vi "AAA Hacker A150-12 THRUST LEVER.vi"() -> ()   [LabVIEW 2020]
uses:
  <instrlib>/Gantner Instruments/Ethernet/Gantner-Instruments HighSpeedPort.llb/e.gate Protocol Type.ctl
  <vilib>/Utility/file.llb/Write Delimited Spreadsheet (string).vi
panel:
  out "Elapsed Time":string
  out "?":dbl[](array[slide]) scale=0.0..1000.0
  out "Temperature 2":dbl[](array[slide]) caption="Thermocouple 1" scale=20.0..50.0
  out "error out 2":errorcluster
  in  "?":bool
  # "Hacker A150-12  -  Motor control"
  # "Temperatures"
  # "Torque"
  # "Vibration"
  # "Power Supply"
  # "Atmospheric\nConditions"
  # "Voltage"
  # "Thrust"
  # "Current"
  # "Battery Data"
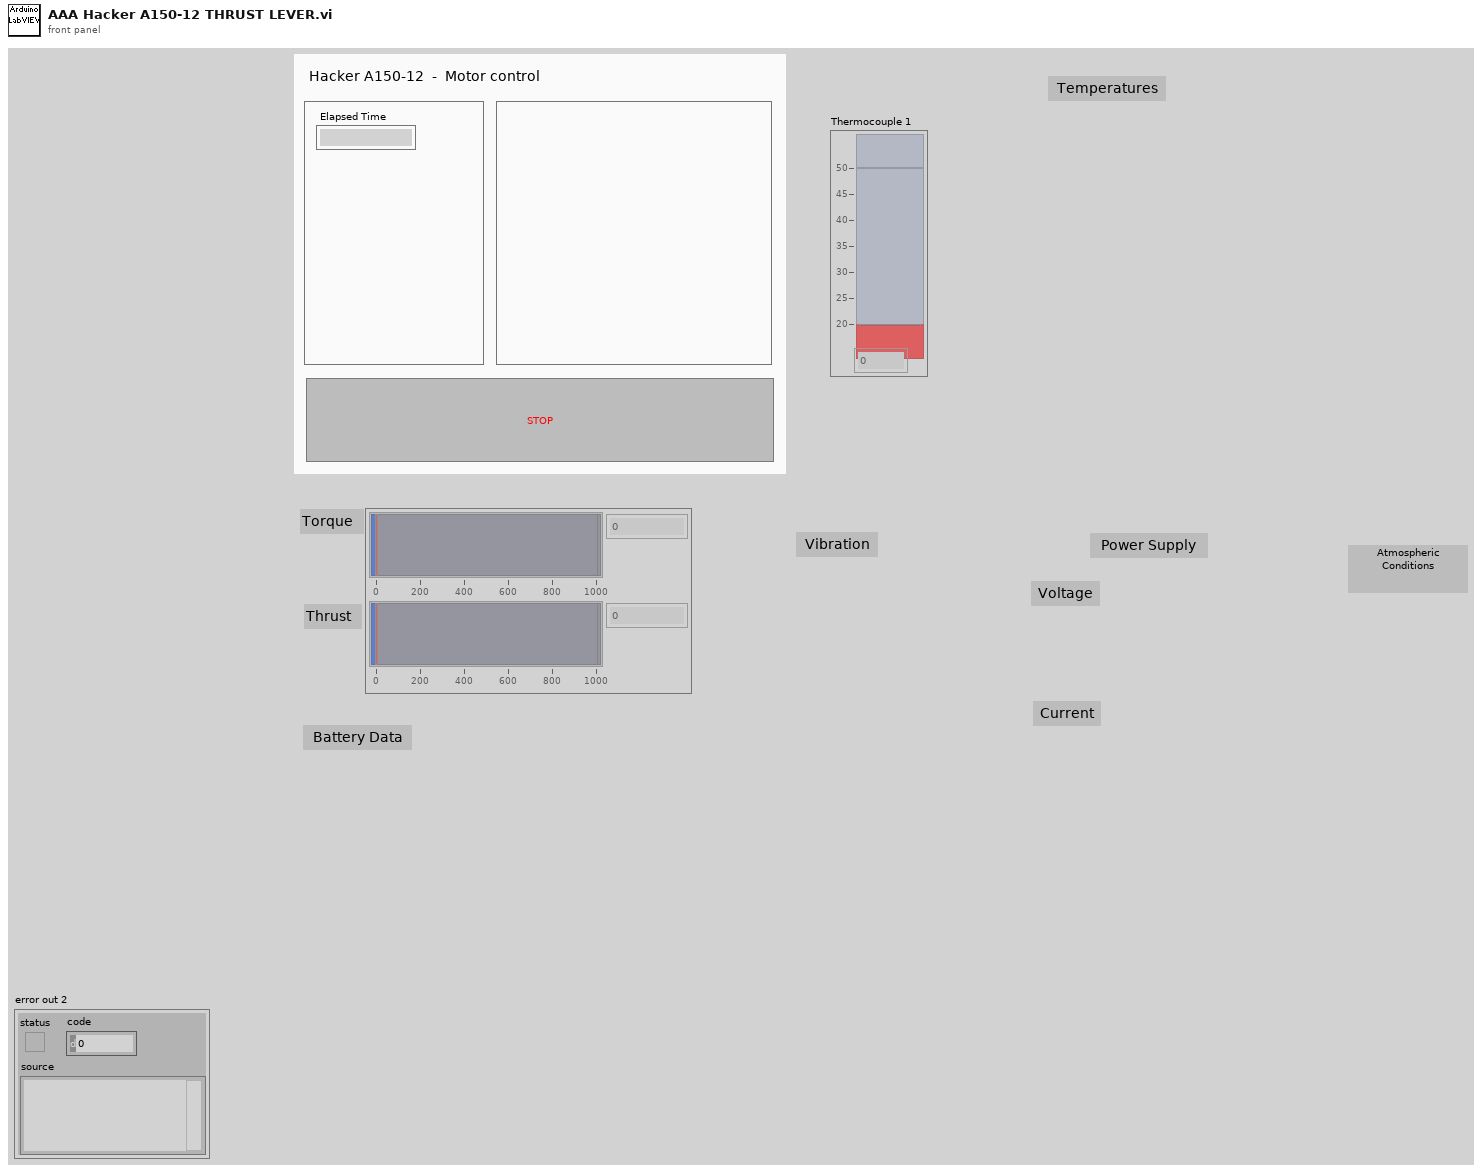
[diagram p1: front panel]
types:
  T1 = typedef "e.gate Protocol Type.ctl" = enum16{"ASCII", "HighspeedPort Online", "HighspeedPort Buffer (giutility.DLL) ", "PostProcessBuffer (giutility.DLL)", "HighspeedPort Online (giutility.DLL)", "Decode UDBF File (giutility.DLL)"}
  T2 = typedef "e.gate Configuration.ctl" = cluster{"connection ID":refnum<k5>, "IPAddress":string, "BufferIndex":i32, "StateMessage":string, "StateCode":i8, "HeaderSize":i32, "BufferSize":i32, "IsBigEndian":i32, "Version":i32, "ChannelCount":i32, "FrameLength":i32, "StartTime":dbl, "dActTimeToSecondFactor":dbl, "StartTimeToDayFactor":dbl, "BufferFillRate":dbl, "SampleRate":dbl, "ChannelData":T3[], "DecodeTimeFormat":string, "SummaryPath":string, "WithCheckSum":i32, "dActTimeDataType":T4, "MaxWriteCount":i32, "MaxReadCount":i32, "TempOffsetRead":i32, "TempLengthRead":i32, "Protocol":T1, "IsSupported":i32, "InputAccessList":i32[], "OutputAccessList":i32[], "DataSource":enum16{"CircleBuffer", "test.con Logger", "test.con Archive"}, "Modules":T5[], "DLL-Handle":T6}
  T3 = typedef "e.gate Channel Data.ctl" = cluster{"VariableName":string, "DataDirection":string, "DataType":string, "DataTypeIndex":T4, "Precision":i16, "FieldLengtht":i16, "ByteCount":i32, "Format":string, "Unit":string, "InputAccessOffset":i32, "OutputAccessOffset":i16, "InputAccessIndex":i16, "OutputAccessIndex":i16, "VarType":string}
  T4 = typedef "e.gate Data Type.ctl" = enum16{"NO", "BOOL", "SINT8", "USINT8", "SINT16", "USINT16", "SINT32", "USINT32", "FLOAT", "SET8", "SET16", "SET32", "DOUBLE", "SINT64", "USINT64", "SET64"}
  T5 = typedef "e.gate Module  Data.ctl" = cluster{"Type":string, "Location":string, "VariablesCount":i16, "UartIndex":i16, "Address":i16, "SystemOffset":i16}
  T6 = typedef "e.gateHSP_DLLhandle.ctl" = cluster{"clientInstance":i32, "connectionInstance":i32, "Is32Bit":bool, "DLL Path":path}
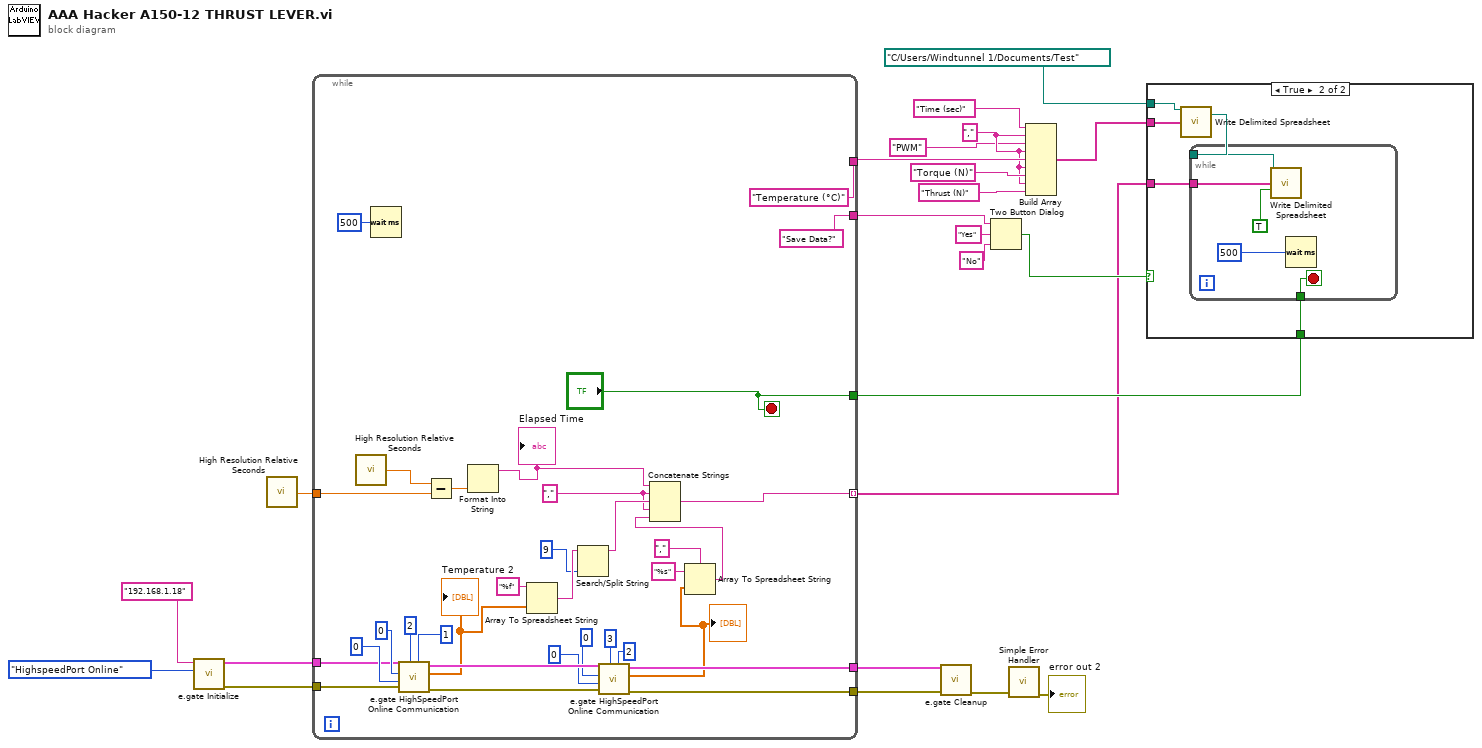
[diagram p0: block diagram]
diagram:
  w2 = "," ("element")
  n1 = call <instrlib>:"e.gate Initialize.vi"("Protocol"=e.gate_Protocol_Type."HighspeedPort Online", "IP Address"="192.168.1.18") -> ("error out"=w18:errorcluster, "e.gate Configuration"=w19:T2)  [unwired: 8 in]
  n2 = call <vilib>:"High Resolution Relative Seconds.vi"() -> ("relative seconds"=w7:dbl)
  n3 = while {
    tunnel: w19 -> [w45]
    tunnel: w18 -> [w44]
    tunnel: [w27] -> w17
    tunnel: [w43] -> w16
    tunnel: ["Save Data?" ("message")] -> w11
    tunnel: ["?"] -> w10
    tunnel: ["Temperature (°C)" ("element")] -> w9
    tunnel: w7 -> [w38]
    tunnel: [w34] -> w8 mode=indexing
    stop <- "?" stop-if-true
    w28 = "," ("string")
    n4 = call <vilib>:"High Resolution Relative Seconds.vi"() -> ("relative seconds"=w39:dbl)
    n5 = Wait (ms)(milliseconds to wait=u32 500) -> ()  [unwired: 1 out]
    n6 = call <instrlib>:"e.gate HighSpeedPort Online Communication.vi"("ReadCount"=1, "ReadIndex"=2, "error in (no error)"=w44, "WriteCount"=0, "WriteIndex"=0, "e.gate Configuration In"=w45) -> ("error out"=w50:errorcluster, "Value"=w40:dbl[], "e.gate Configuration Out"=w51:T2)  [unwired: 3 in]
    "Temperature 2" <- w40
    n7 = Subtract(x=w39, y=w38) -> (x-y=w37:dbl)
    n8 = Format Into String(w37) -> (resulting string=w25:string)  [unwired: 3 in, 1 out]
    "Elapsed Time" <- w25
    n9 = Array To Spreadsheet String(array=w40, 3:"%f" ("format string")) -> (spreadsheet string=w31:string)  [unwired: 1 in]
    n10 = Search/Split String(string=w31, offset (0)=9) -> (substring before match=w30:string)  [unwired: 1 in, 2 out]
    n11 = call <instrlib>:"e.gate HighSpeedPort Online Communication.vi"("ReadCount"=2, "ReadIndex"=3, "error in (no error)"=w50, "WriteCount"=0, "WriteIndex"=0, "e.gate Configuration In"=w51) -> ("error out"=w43:errorcluster, "Value"=w24:dbl[], "e.gate Configuration Out"=w27:T2)  [unwired: 3 in]
    "?" <- w24
    n12 = Array To Spreadsheet String(delimiter (Tab)=",", array=w24, 3:"%s" ("format string")) -> (spreadsheet string=w32:string)
    n13 = Concatenate Strings(w25, w28, w30, w28, w32) -> (w34:string)
  }
  n14 = call <instrlib>:"e.gate Cleanup.vi"("error in (no error)"=w16, "e.gate Configuration"=w17) -> ("error out"=w23:errorcluster)  [unwired: 9 in]
  n15 = Two Button Dialog(message=w11, 1:"No" ("F button name (\"Cancel\")"), 2:"Yes" ("T button name (\"OK\")")) -> (T button?=w14:bool)
  n16 = call <vilib>:"Simple Error Handler.vi"("error in (no error)"=w23) -> ("error out"=→"error out 2":errorcluster)  [unwired: 4 in, 4 out]
  n17 = Build Array("Time (sec)" ("element"), w2, "PWM" ("element"), w2, w9, w2, "Torque (N)" ("element"), w2, "Thrust (N)" ("element")) -> (w15:string[])
  n18 = case shown="True" w14 {
    tunnel: w15 -> [_ w60]
    tunnel: w10 -> [_ w59]
    tunnel: w8 -> [_ w58]
    tunnel: path "C:/Users/Windtunnel 1/Documents/Test" ("file path (dialog if empty) 2") -> [_ w57]
    frame False {
    }
    frame True {
      n19 = call-poly <vilib>:"Write Delimited Spreadsheet.vi"("file path (dialog if empty)"=w57, "1D data"=w60) -> ("new file path (Not A Path if cancelled)"=w61:path)  [unwired: 12 in, 1 out]
      n20 = while {
        tunnel: w61 -> [w66]
        tunnel: w59 -> [w63]
        tunnel: w58 -> [w62]
        stop <- w63 stop-if-true
        n21 = call-poly <vilib>:"Write Delimited Spreadsheet.vi"("file path (dialog if empty)"=w66, "1D data"=w62, "append to file? (new file:F)"=TRUE) -> ()  [unwired: 11 in, 2 out]
        n22 = Wait (ms)(milliseconds to wait=u32 500) -> ()  [unwired: 1 out]
      }
    }
  }
